vi "OAT Convert Phase (1 channel).vi"(6 "input unit in degree?":bool, 7 "reset (TRUE)":bool=TRUE, 10 "desired phase setting":T1, 11 "phase in (rad)":dbl[][](array[numeric]) format="%.2f") -> (3 "phase out":dbl[][](array[numeric]) format="%.2f")   [LabVIEW 2017]
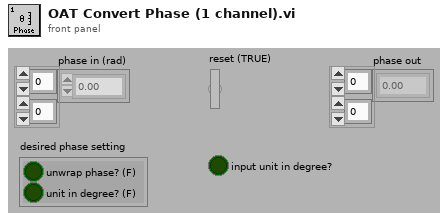
[diagram p1: front panel]
types:
  T1 = cluster{"unwrap phase? (F)":bool, "unit in degree? (F)":bool}
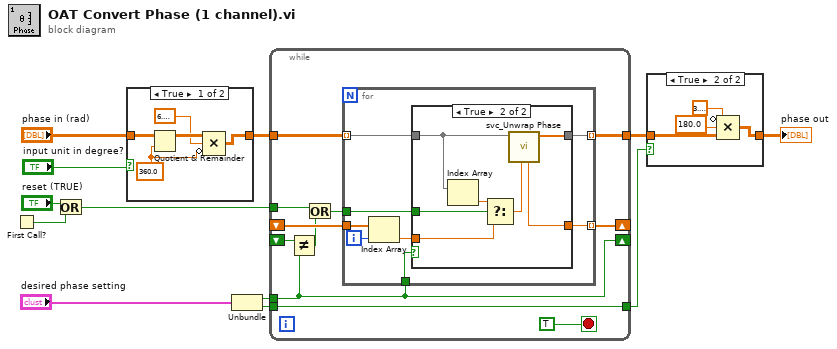
[diagram p0: block diagram]
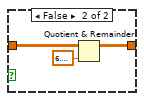
[diagram p3: hidden frame]
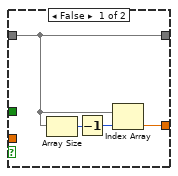
[diagram p4: hidden frame]
diagram:
  n1 = First Call?() -> (First Call?: T/F=w7:bool)
  n2 = Or(x="reset (TRUE)", y=w7) -> (x .or. y?=w6:bool)
  n3 = case shown="True" "input unit in degree?" {
    tunnel: "phase in (rad)" -> [w17 w19]
    tunnel: [w13 w18] -> w9
    frame True {
      w14 = 360.0
      n4 = Quotient & Remainder(x=w17, y=w14) -> (x-y*floor(x/y)=w16:dbl[][])  [unwired: 1 out]
      n5 = Compound Arithmetic op=MULTIPLY(w16, 6.283185307179586, invert w14) -> (w13:dbl[][])
    }
    frame False {
      n6 = Quotient & Remainder(x=w19, y=6.283185307179586) -> (x-y*floor(x/y)=w18:dbl[][])  [unwired: 1 out]
    }
  }
  n7 = Unbundle("desired phase setting") -> ("unwrap phase? (F)"=w12:bool, "unit in degree? (F)"=w11:bool)
  n8 = while {
    tunnel: [w22] -> w4
    tunnel: w12 -> [w27]
    tunnel: w11 -> [w21]
    tunnel: w9 -> [w31]
    shift-right: [w28] -> _
    shift-left: _ -> [w29]
    tunnel: w6 -> [w25]
    shift-right: [w27] -> _
    shift-left: _ -> [w23]
    tunnel: [w21] -> w2
    stop <- TRUE stop-if-true
    n9 = Not Equal?(x=w23, y=w27) -> (x != y?=w26:bool)
    n10 = Or(x=w25, y=w26) -> (x .or. y?=w24:bool)
    n11 = for {
      tunnel: [w36] -> w22 mode=indexing
      tunnel: w27 -> [w39]
      tunnel: w31 -> [w38] mode=indexing
      tunnel: w29 -> [w34]
      tunnel: w24 -> [w35]
      tunnel: [w37] -> w28 mode=indexing
      i -> [w32]
      n12 = Index Array(array=w34, index=w32) -> (element=w33:dbl)
      n13 = case shown="True" w39 {
        tunnel: [w43 w45] -> w36
        tunnel: w38 -> [w43 w47]
        tunnel: [w40 w44] -> w37
        tunnel: w33 -> [_ w49]
        tunnel: w35 -> [_ w48]
        frame False {
          n14 = Array Size(array=w43) -> (size(s)=w42:i32)
          n15 = Decrement(x=w42) -> (x-1=w41:i32)
          n16 = Index Array(array=w43, index=w41) -> (element=w40:dbl)
        }
        frame True {
          n17 = Index Array(array=w47) -> (element=w50:dbl)  [unwired: 1 in]
          n18 = Select(t=w50, s=w48, f=w49) -> (s? t:f=w46:dbl)
          n19 = call <vilib>:"svc_Unwrap Phase.vi"("start phase"=w46, "phase in"=w47) -> ("phase out"=w45:dbl[], "end phase"=w44:dbl)  [unwired: 8 in]
        }
      }
    }
  }
  n20 = case shown="True" w2 {
    tunnel: w4 -> [w51 w53]
    tunnel: [w51 w52] -> w3
    frame False {
    }
    frame True {
      n21 = Compound Arithmetic op=MULTIPLY(invert 3.141592653589793, 180.0, w53) -> (w52:dbl[][])
    }
  }
  "phase out" <- w3
